vi "BrakeRelease.vi"(0 "Universal Robot.lvclass in":refnum<class "Universal Robot.lvclass">, 5 "error in (no error)":errorcluster) -> (14 "Universal Robot.lvclass out":refnum<class "Universal Robot.lvclass">, 19 "error out":errorcluster)   [LabVIEW 2019, in "Universal Robot.lvclass"]
uses:
  Universal Robot.lvclass
  Universal Robot.lvclass/Universal Robot.ctl
  RobotMode.ctl
  Client Interfaces/Dashboard Server/Dashboard Server.lvclass
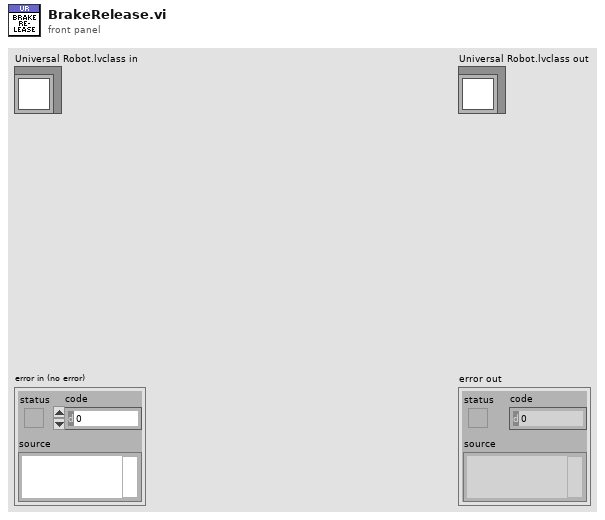
[diagram p1: front panel]
types:
  T1 = typedef "Universal Robot.lvclass/RobotMode.ctl" = enum16{"INVALID", "NO_CONTROLLER", "DISCONNECTED", "CONFIRM_SAFETY", "BOOTING", "POWER_OFF", "POWER_ON", "IDLE", "BACKDRIVE", "RUNNING"}
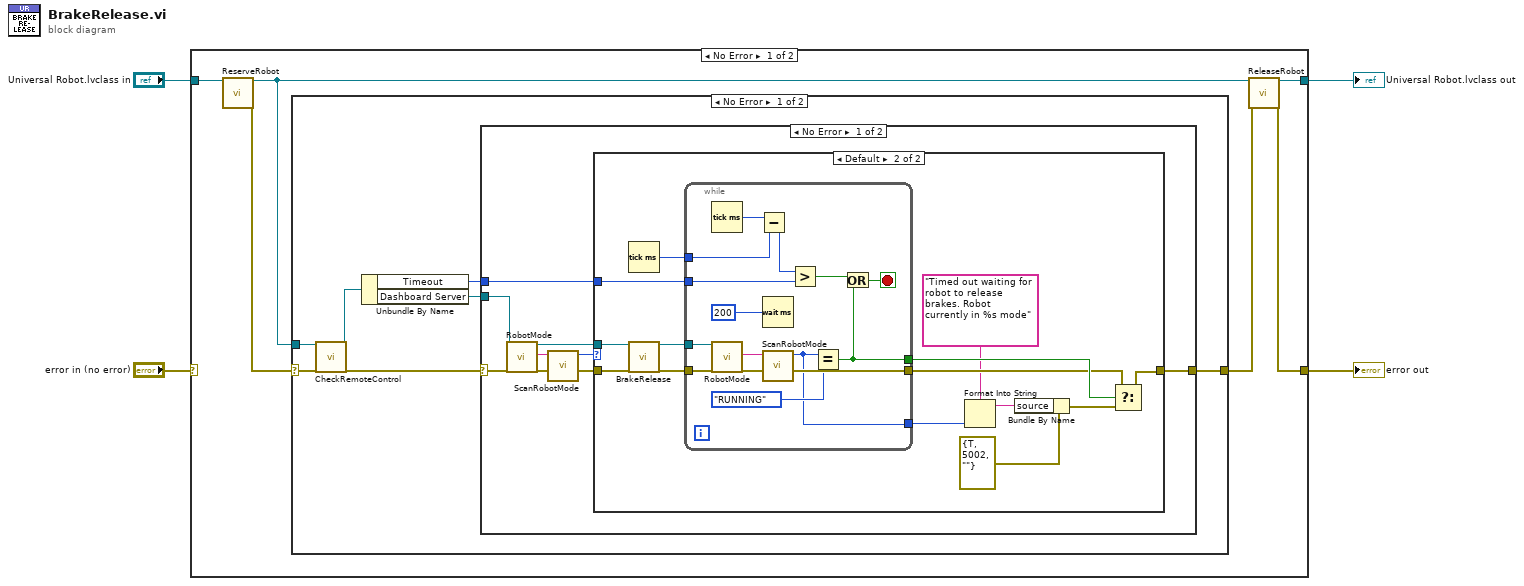
[diagram p0: block diagram]
diagram:
  n1 = case shown="No Error" "error in (no error)" {
    selector: "error in (no error)" -> [_ w58]
    tunnel: [w6 w58] -> w3
    tunnel: "Universal Robot.lvclass in" -> [w10 w57]
    tunnel: [w8 w57] -> w1
    frame No Error {
      n2 = call "ReserveRobot.vi"("Universal Robot.lvclass in"=w10) -> ("Universal Robot.lvclass out"=w9:refnum<class "Universal Robot.lvclass">, "error out"=w5:errorcluster)  [unwired: 17 in]
      n3 = case shown="No Error" w5 {
        selector: w5 -> [w11 w56]
        tunnel: w9 -> [w13 _]
        tunnel: [w12 w56] -> w7
        frame No Error {
          n4 = call-dynamic "CheckRemoteControl.vi"("Universal Robot.lvclass in"=w13, "error in (no error)"=w11) -> ("Universal Robot.lvclass out"=w17:refnum<class "Universal Robot.lvclass">, "error out"=w14:errorcluster)  [unwired: 16 in]
          n5 = Unbundle By Name(w17) -> ("Timeout"=w15:u32, "Dashboard Server"=w16:refnum<class "Dashboard Server.lvclass">)
          n6 = case shown="No Error" w14 {
            selector: w14 -> [w20 w55]
            tunnel: [w25 w55] -> w12
            tunnel: w16 -> [w24 _]
            tunnel: w15 -> [w23 _]
            frame No Error {
              n7 = call-dynamic "RobotMode.vi"("DashboardServer in"=w24, "error in (no error)"=w20) -> ("DashboardServer out"=w21:refnum<class "Dashboard Server.lvclass">, "robotMode"=w19:string, "error out"=w22:errorcluster)  [unwired: 15 in]
              n8 = call "ScanRobotMode.vi"("robotMode in"=w19) -> ("robotMode out"=w18:T1)  [unwired: 10 in]
              n9 = case shown="Default" w18 {
                tunnel: [w26 w36] -> w25
                tunnel: w22 -> [w26 w29]
                tunnel: w21 -> [_ w30]
                tunnel: w23 -> [_ w40]
                frame "RUNNING" {
                  # "Robot is already running"
                }
                frame Default {
                  n10 = Tick Count (ms)() -> (millisecond timer value=w39:u32)
                  n11 = call-dynamic "BrakeRelease.vi"("DashboardServer in"=w30, "error in (no error)"=w29) -> ("DashboardServer out"=w28:refnum<class "Dashboard Server.lvclass">, "error out"=w27:errorcluster)  [unwired: 16 in]
                  n12 = while {
                    tunnel: w28 -> [w53]
                    tunnel: w27 -> [w54]
                    tunnel: [w52] -> w37
                    tunnel: w40 -> [w50]
                    tunnel: w39 -> [w49]
                    tunnel: [w44] -> w38
                    tunnel: [w41] -> w35
                    stop <- w45 stop-if-true
                    n13 = Tick Count (ms)() -> (millisecond timer value=w48:u32)
                    n14 = call-dynamic "RobotMode.vi"("DashboardServer in"=w53, "error in (no error)"=w54) -> ("robotMode"=w43:string, "error out"=w52:errorcluster)  [unwired: 15 in, 1 out]
                    n15 = Subtract(x=w48, y=w49) -> (x-y=w47:u32)
                    n16 = Wait (ms)(milliseconds to wait=u32 200) -> ()  [unwired: 1 out]
                    n17 = call "ScanRobotMode.vi"("robotMode in"=w43) -> ("robotMode out"=w41:T1)  [unwired: 10 in]
                    n18 = Greater?(x=w47, y=w50) -> (0:w46:bool)
                    n19 = Equal?(x=w41, y=RobotMode."RUNNING") -> (x = y?=w44:bool)
                    n20 = Or(x=w46, y=w44) -> (x .or. y?=w45:bool)
                  }
                  n21 = Format Into String(format string="Timed out waiting for robot to release brakes. Robot currently in %s mode", w35) -> (resulting string=w33:string)  [unwired: 2 in, 1 out]
                  n22 = Bundle By Name(cluster=errorcluster {"status"=TRUE, "code"=5002, "source"=""} ("error constant"), "source"=w33) -> (w32:errorcluster)
                  n23 = Select(t=w37, s=w38, f=w32) -> (s? t:f=w36:errorcluster)
                }
              }
            }
            frame Error {
            }
          }
        }
        frame Error {
        }
      }
      n24 = call "ReleaseRobot.vi"("Universal Robot.lvclass in"=w9, "error in (no error)"=w7) -> ("Universal Robot.lvclass out"=w8:refnum<class "Universal Robot.lvclass">, "error out"=w6:errorcluster)  [unwired: 16 in]
    }
    frame Error {
    }
  }
  "error out" <- w3
  "Universal Robot.lvclass out" <- w1
